vi "readCommandStart.vi"(8 "error in (no error)":errorcluster, 10 "Parser":refnum<class "U8ArrayParserAutoIndexing.lvclass">, 11 "M1M3SAL in":refnum<class "M1M3SAL.lvclass">) -> (0 "error out":errorcluster, 2 "CommandStart":variant, 3 "M1M3SAL out":refnum<class "M1M3SAL.lvclass">)   [LabVIEW 2016, in "M1M3SupportCommunicator.lvlib" / "M1M3SAL.lvclass"]
uses:
  M1M3SAL.lvclass
  Common_RT_Utilities/U8ArrayParserAutoIndexing/U8ArrayParserAutoIndexing.lvclass
  DataTypes/Topics/CommandStart.ctl
  DataTypes/Topics/Parts/CommandId.ctl
  DataTypes/Topics/M1M3SupportTopics.lvlib
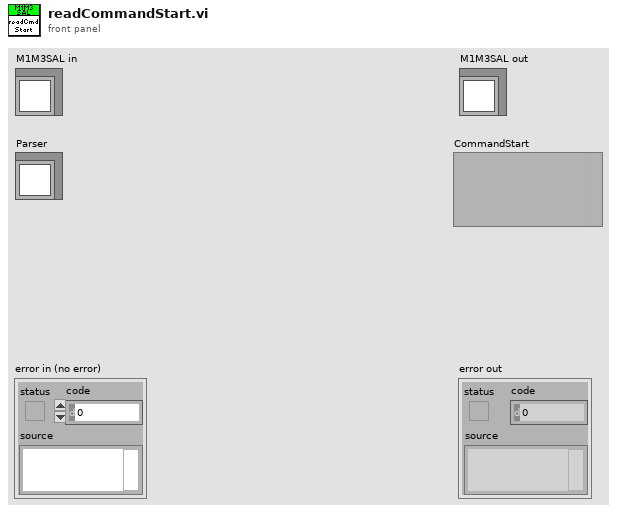
[diagram p1: front panel]
types:
  T1 = typedef "M1M3SupportTopics.lvlib/CommandStart.ctl" = cluster{"CommandId":T2, "Start":bool, "SettingToApply":string}
  T2 = typedef "M1M3SupportTopics.lvlib/CommandId.ctl" = i32
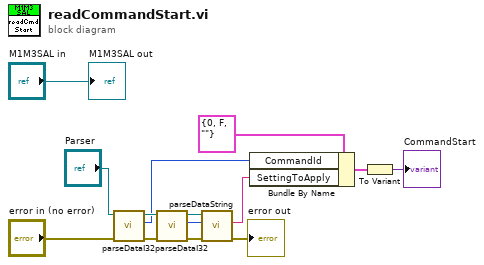
[diagram p0: block diagram]
diagram:
  n1 = call "parseDataI32.vi"("error in (no error)"="error in (no error)", "U8ArrayParserAutoIndexing in"="Parser") -> ("error out"=w2:errorcluster, "Data"=w1:i32, "U8ArrayParserAutoIndexing out"=w3:refnum<class "U8ArrayParserAutoIndexing.lvclass">)  [unwired: 7 in]
  n2 = call "parseDataI32.vi"("error in (no error)"=w2, "U8ArrayParserAutoIndexing in"=w3) -> ("error out"=w7:errorcluster, "Data"=w10:i32, "U8ArrayParserAutoIndexing out"=w9:refnum<class "U8ArrayParserAutoIndexing.lvclass">)  [unwired: 7 in]
  n3 = call "parseDataString.vi"("error in (no error)"=w7, "Length"=w10, "U8ArrayParserAutoIndexing in"=w9) -> ("error out"=→"error out":errorcluster, "Data"=w8:string)  [unwired: 6 in, 1 out]
  n4 = Bundle By Name(cluster=T1 {"CommandId"=0, "Start"=FALSE, "SettingToApply"=""} ("CommandStart"), "CommandId"=w1, "SettingToApply"=w8) -> (w12:T1)
  n5 = To Variant(anything=w12) -> (Variant=→"CommandStart":variant)
  "M1M3SAL out" <- "M1M3SAL in"
